vi "剖面管理.vi"() -> ()   [LabVIEW 2010]
panel:
  in  "Numeric":dbl
  in  "当前连接的控制器":string
  in  "读取剖面列表":bool
  in  "返回":bool
  in  "删除剖面":bool
  in  "执行选中剖面":bool
  in  "Listbox":i32(listbox)
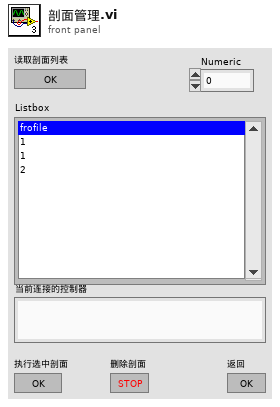
[diagram p1: front panel]
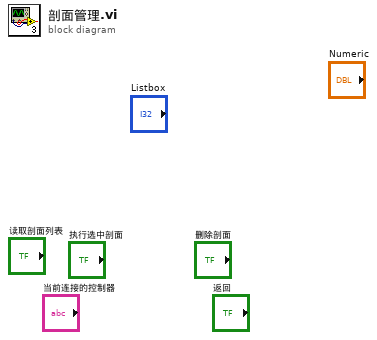
[diagram p0: block diagram]
diagram:
